vi "固定站CODCr测量流程.vi"(11 "控制命令":T1(ring)) -> ()   [LabVIEW 2016, in "CODCr库.lvlib"]
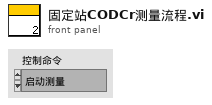
[diagram p1: front panel]
types:
  T1 = enum16{"启动测量", "标样核查", "零点核查", "跨度核查", "空白测试", "平行样测试", "加标回收", "空白校准", "标样校准", "初始化（清洗）", "停止测试", "仪器重启", "校时", "模式设置", "测量间隔设置"}
  T2 = cluster{"命令":string, "测量模式":enum16{"水样测量", "标样核查", "零点核查", "跨度核查", "空白测试", "加标回收", "平行样", "校零", "校标"}, "CODCr量程切换":enum32{"H", "L", "AUTO"}}
  T3 = cluster{"仪器":enum16{"", "氨氮", "总磷", "总氮", "CODMn", "CODCr"}, "启动命令":enum16{"启动水样流程", "启动加标流程", "排液", "停止", "柱塞泵启动"}}
  T4 = cluster{"时间标识":timestamp, "参数":string, "日志信息":string, "流程参数":string}
  T5 = enum16{"水样测量", "标样核查", "零点核查", "跨度核查", "空白测试", "加标回收", "平行样", "校零", "校标"}
  T6 = cluster{"命令":string, "测量模式":enum16{"水样测量", "标样核查", "零点核查", "跨度核查", "空白测试", "加标回收", "平行样", "校零", "校标"}, "CODMn量程切换":enum32{"H", "L", "AUTO"}}
  T7 = cluster{"时间标识":timestamp, "设备":string, "日志信息":string, "流程参数":string}
  T8 = cluster{"系统时间":timestamp, "工作状态":u16, "测量模式":u16, "告警代码":u16, "故障代码":u16, "日志代码":u16, "软件版本":u16, "F0":sgl, "F1":sgl, "F2":sgl, "F3":sgl, "T":sgl, "H":sgl, "id":u16, "flowid":u16, "量程":u16}
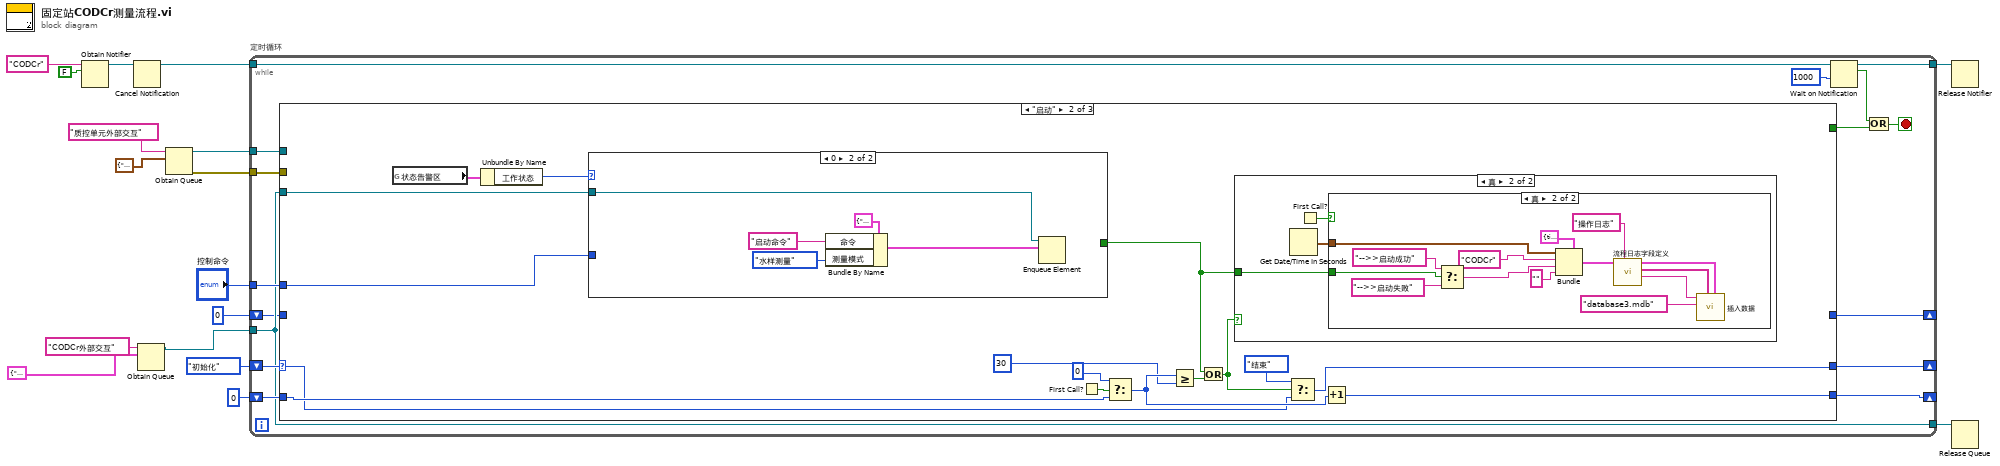
[diagram p0: block diagram]
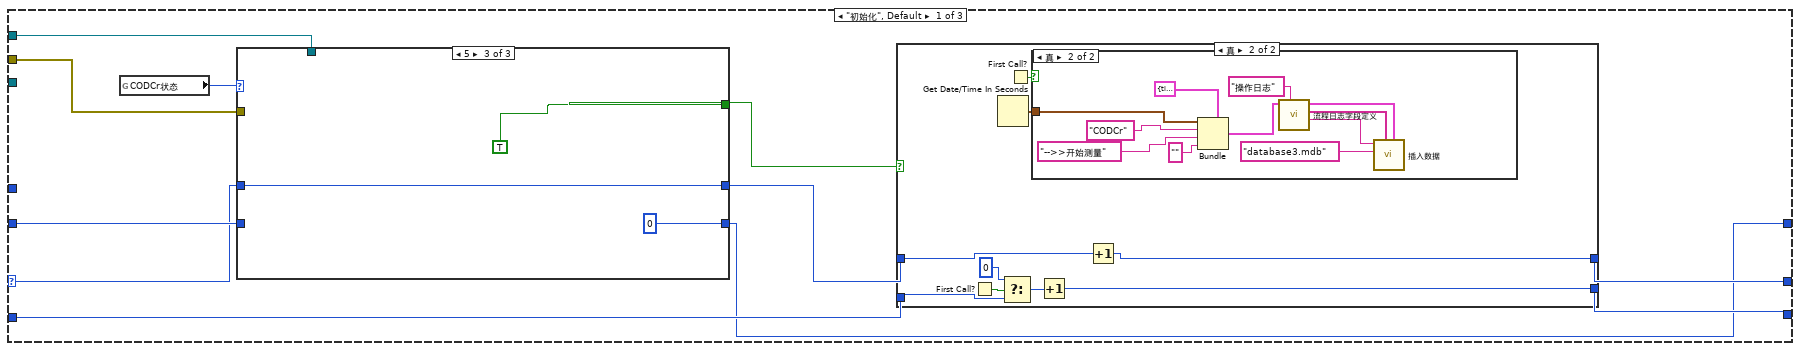
[diagram p2: hidden frame]
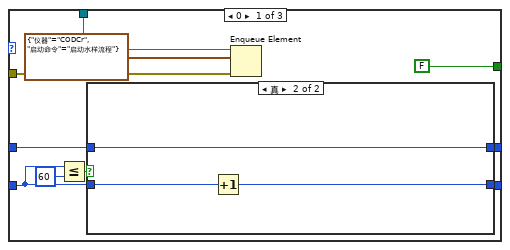
[diagram p5: hidden frame]
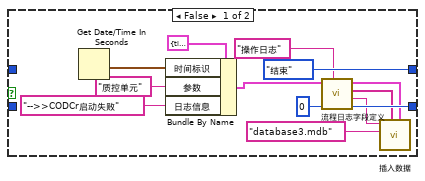
[diagram p6: hidden frame]
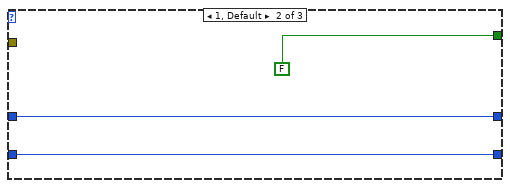
[diagram p7: hidden frame]
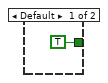
[diagram p10: hidden frame]
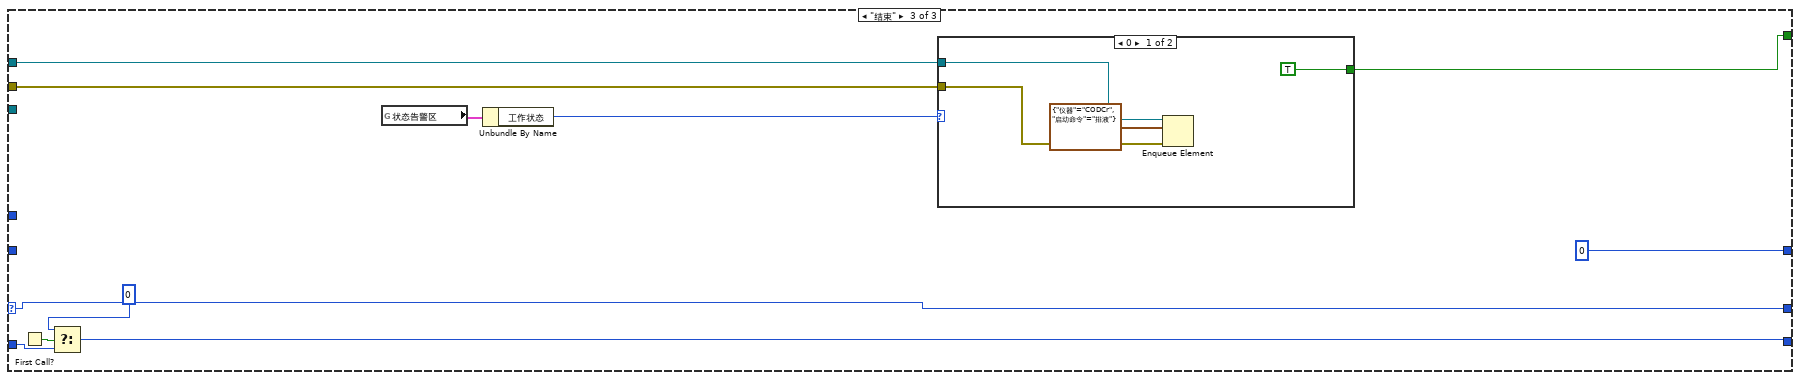
[diagram p11: hidden frame]
diagram:
  n1 = Obtain Notifier(name (unnamed)="CODCr" ("名称（未命名）"), notification data type=FALSE) -> (notifier out=w15:refnum<notifier>)  [unwired: 2 in, 2 out]
  n2 = Cancel Notification(0:w15) -> (8:w14:refnum<notifier>)  [unwired: 1 in, 2 out]
  n3 = Obtain Queue(name (unnamed)="CODCr外部交互" ("名称（未命名）"), element data type=T2 {"命令"="启动命令", "测量模式"=enum."水样测量", "CODCr量程切换"=enum."AUTO"} ("元素")) -> (queue out=w1:refnum<queue>)  [unwired: 3 in, 2 out]
  n4 = Obtain Queue(name (unnamed)="质控单元外部交互" ("名称（未命名）"), element data type=T3 {"仪器"=enum."氨氮", "启动命令"=enum."启动水样流程"} ("元素")) -> (queue out=w6:refnum<queue>, error out=w5:errorcluster)  [unwired: 3 in, 1 out]
  n5 = while "定时循环" {
    tunnel: w1 -> [w22]
    tunnel: w14 -> [w33]
    tunnel: "控制命令" -> [w28]
    shift-right: [w27] -> _
    shift-left: enum16{"初始化", "启动", "结束"}."初始化" -> [w29]
    shift-right: [w25] -> _
    shift-left: 0 -> [w26]
    tunnel: [w23] -> w10
    tunnel: [w22] -> w11
    tunnel: w6 -> [w21]
    tunnel: w5 -> [w20]
    shift-right: [w18] -> _
    shift-left: 0 -> [w19]
    stop <- w30 stop-if-true
    n6 = case shown="\"启动\"" w29 {
      selector: w29 -> [w36 w104 w147]
      tunnel: w28 -> [_ w113 _]
      tunnel: w22 -> [_ w112 _]
      tunnel: [w44 w105 w147] -> w27
      tunnel: w26 -> [w43 w109 w144]
      tunnel: [w42 w108 w143] -> w25
      tunnel: [_ _ w140] -> w24
      tunnel: w21 -> [w40 _ w142]
      tunnel: w20 -> [w39 _ w141]
      tunnel: w19 -> [w38 _ _]
      tunnel: [w37 _ 0] -> w18
      frame "初始化", Default {
        n7 = global read "CODCr外部API.vi" "CODCr状态"() -> (w34:u16)
        n8 = case shown="5" w34 {
          tunnel: [FALSE ("s") FALSE ("s") TRUE ("s")] -> w41
          tunnel: w40 -> [w75 _ _]
          tunnel: w39 -> [w74 _ _]
          tunnel: w38 -> [w72 w92 _]
          tunnel: [w69 w92 0] -> w37
          tunnel: w36 -> [w68 w93 w96]
          tunnel: [w67 w93 w96] -> w35
          frame 0 {
            n9 = Less Or Equal?(x=w72, y=60) -> (x <= y?=w70:bool)
            n10 = case shown="真" w70 {
              tunnel: w72 -> [_ w91]
              tunnel: [0 w90] -> w69
              tunnel: w68 -> [_ w89]
              tunnel: [enum16{"初始化", "启动", "结束"}."结束" w89] -> w67
              frame False {
                n11 = Get Date/Time In Seconds() -> (seconds since 1Jan1904=w84:timestamp)
                n12 = Bundle By Name(cluster=T4 {"时间标识"=timestamp(0 s since 1904-01-01), "参数"="", "日志信息"="", "流程参数"=""} ("data in"), "时间标识"=w84, "参数"="质控单元" ("设备"), "日志信息"="-->>CODCr启动失败") -> (w78:T4)
                n13 = call "流程日志字段定义.vi"("table输入"="操作日志", "data in"=w78) -> ("table输出"=w81:string, "columns"=w82:string[], "data out"=w83:T7)  [unwired: 7 in]
                n14 = call "插入数据.vi"("data"=w83, "columns"=w82, "database"="database3.mdb", "table"=w81) -> ()  [unwired: 7 in, 1 out]
              }
              frame True {
                n15 = Increment(x=w91) -> (x+1=w90:i32)
              }
            }
            n16 = Enqueue Element(queue=w75, element=T3 {"仪器"=enum."CODCr", "启动命令"=enum."启动水样流程"} ("元素"), error in (no error)=w74) -> ()  [unwired: 1 in, 3 out]
          }
          frame 1, Default {
          }
          frame 5 {
          }
        }
        n17 = case shown="真" w41 {
          tunnel: w35 -> [w46 w53]
          tunnel: [w46 w52] -> w44
          tunnel: w43 -> [w45 w50]
          tunnel: [w45 w47] -> w42
          frame False {
          }
          frame True {
            n18 = First Call?() -> (First Call?: T/F=w51:bool)
            n19 = Get Date/Time In Seconds() -> (seconds since 1Jan1904=w55:timestamp)
            n20 = Select(t=0, s=w51, f=w50) -> (s? t:f=w48:i32)
            n21 = First Call?() -> (First Call?: T/F=w54:bool)
            n22 = case shown="真" w54 {
              tunnel: w55 -> [_ w63]
              frame False {
              }
              frame True {
                n23 = Bundle(cluster=T4 {"时间标识"=timestamp(0 s since 1904-01-01), "参数"="", "日志信息"="", "流程参数"=""} ("data in"), "时间标识"=w63, "参数"="CODCr" ("设备"), "日志信息"="-->>开始测量", "流程参数"="" ("table输入")) -> (w56:T4)
                n24 = call "流程日志字段定义.vi"("table输入"="操作日志", "data in"=w56) -> ("table输出"=w59:string, "columns"=w58:string[], "data out"=w57:T7)  [unwired: 7 in]
                n25 = call "插入数据.vi"("data"=w57, "columns"=w58, "database"="database3.mdb", "table"=w59) -> ()  [unwired: 7 in, 1 out]
              }
            }
            n26 = Increment(x=w48) -> (x+1=w47:i32)
            n27 = Increment(x=w53) -> (x+1=w52:enum16{"初始化", "启动", "结束"})
          }
        }
      }
      frame "启动" {
        n28 = global read "CODcr全局变量.vi" "状态告警区"() -> (w99:T8)
        n29 = Unbundle By Name(w99) -> ("工作状态"=w98:u16)
        n30 = case shown="0" w98 {
          tunnel: w113 -> [_ _]
          tunnel: w112 -> [_ w136]
          tunnel: [TRUE _] -> w100
          frame Default {
          }
          frame 0 {
            n31 = Bundle By Name(cluster=T6 {"命令"="启动命令", "测量模式"=enum."水样测量", "CODMn量程切换"=enum."AUTO"} ("元素"), "命令"="启动命令", "测量模式"=T5."水样测量") -> (w133:T6)
            n32 = Enqueue Element(queue=w136, element=w133) -> ()  [unwired: 2 in, 3 out]
          }
        }
        n33 = First Call?() -> (First Call?: T/F=w111:bool)
        n34 = Select(t=0, s=w111, f=w109) -> (s? t:f=w107:i32)
        n35 = Greater Or Equal?(x=w107, y=30) -> (x >= y?=w103:bool)
        n36 = Or(x=w100, y=w103) -> (x .or. y?=w101:bool)
        n37 = case shown="真" w101 {
          tunnel: w100 -> [_ w114]
          frame False {
          }
          frame True {
            n38 = Get Date/Time In Seconds() -> (seconds since 1Jan1904=w115:timestamp)
            n39 = First Call?() -> (First Call?: T/F=w116:bool)
            n40 = case shown="真" w116 {
              tunnel: w115 -> [_ w119]
              tunnel: w114 -> [_ w130]
              frame False {
              }
              frame True {
                n41 = Select(t="-->>启动成功" ("日志信息"), s=w130, f="-->>启动失败" ("日志信息")) -> (s? t:f=w117:string)
                n42 = Bundle(cluster=T4 {"时间标识"=timestamp(0 s since 1904-01-01), "参数"="", "日志信息"="", "流程参数"=""} ("data in"), "时间标识"=w119, "参数"="CODCr" ("设备"), "日志信息"=w117, "流程参数"="" ("table输入")) -> (w125:T4)
                n43 = call "流程日志字段定义.vi"("table输入"="操作日志", "data in"=w125) -> ("table输出"=w122:string, "columns"=w121:string[], "data out"=w120:T7)  [unwired: 7 in]
                n44 = call "插入数据.vi"("data"=w120, "columns"=w121, "database"="database3.mdb", "table"=w122) -> ()  [unwired: 7 in, 1 out]
              }
            }
          }
        }
        n45 = Select(t=enum16{"初始化", "启动", "结束"}."结束", s=w101, f=w104) -> (s? t:f=w105:enum16{"初始化", "启动", "结束"})
        n46 = Increment(x=w107) -> (x+1=w108:i32)
      }
      frame "结束" {
        n47 = First Call?() -> (First Call?: T/F=w146:bool)
        n48 = Select(t=0, s=w146, f=w144) -> (s? t:f=w143:i32)
        n49 = global read "CODcr全局变量.vi" "状态告警区"() -> (w138:T8)
        n50 = Unbundle By Name(w138) -> ("工作状态"=w137:u16)
        n51 = case shown="0" w137 {
          tunnel: w142 -> [w150 _]
          tunnel: w141 -> [w149 _]
          tunnel: [TRUE _] -> w140
          frame 0 {
            n52 = Enqueue Element(queue=w150, element=T3 {"仪器"=enum."CODCr", "启动命令"=enum."排液"} ("元素"), error in (no error)=w149) -> ()  [unwired: 1 in, 3 out]
          }
          frame 1, Default {
          }
        }
      }
    }
    n53 = Wait on Notification(notifier=w33, timeout in ms (-1)=1000 ("超时毫秒(-1)")) -> (notifier out=w23:refnum<notifier>, notification=w31:bool)  [unwired: 2 in, 2 out]
    n54 = Or(x=w31, y=w24) -> (x .or. y?=w30:bool)
  }
  n55 = Release Notifier(notifier=w10) -> ()  [unwired: 2 in, 3 out]
  n56 = Release Queue(queue=w11) -> ()  [unwired: 2 in, 3 out]
